vi "Resize Image.vi"(8 "error in (no error)":errorcluster, 11 "Save Image in":refnum<class "Save Image.lvclass">) -> (0 "error out":errorcluster, 3 "Save Image out":refnum<class "Save Image.lvclass">)   [LabVIEW 2018, in "Save Image.lvclass"]
uses:
  Save Image.lvclass
  Interface/Interface.lvclass
  <userlib>/gfitsio/gfitsio.lvlib
  <userlib>/gfitsio/cfitsio-bitpix.ctl
  Simulated_Header/Simulated_Header.lvclass
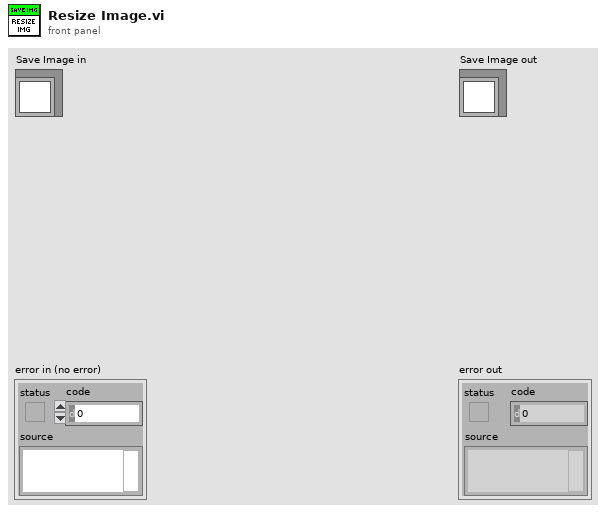
[diagram p1: front panel]
types:
  T1 = typedef "gfitsio.lvlib/cfitsio-bitpix.ctl" = i32
  T2 = cluster{"PREAMP":u16, "READOUT_RATE":u16, "EM_GAIN":u16, "VBIN":u16, "INITIAL_LINE":u16, "INITIAL_COLUMN":u16, "FINAL_LINE":u16, "FINAL_COLUMN":u16, "TRIGGER_MODE":u16, "HBIN":u16, "SHUTTER_TTL":u16, "SHUTTER_MODE":u16, "SHUTTER_OPENING_TIME":u16, "SHUTTER_CLOSING_TIME":u16, "VERTICAL_SHIFT_SPEED":u16, "READ_MODE":u16, "FRAME_TRANSFER":bool, "VERTICAL_CLOCK_VOLTAGE":u16, "ACQUISITION_MODE":u16, "AD_CHANNEL":u16, "EM_MODE":u16}
  T3 = typedef "gfitsio.lvlib/gfitsio-refnum.ctl" = refnum<k1>
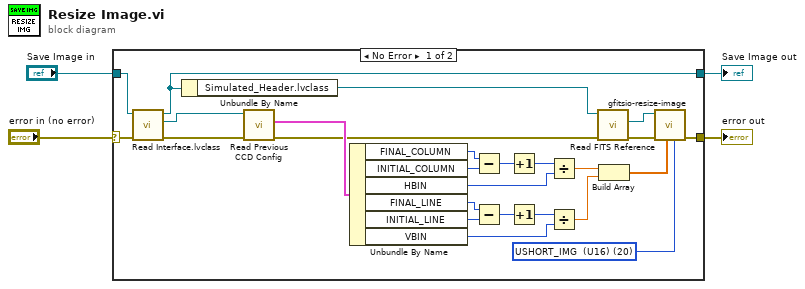
[diagram p0: block diagram]
diagram:
  n1 = case shown="No Error" "error in (no error)" {
    selector: "error in (no error)" -> [w8 w31]
    tunnel: [w12 w31] -> w3
    tunnel: [w5 w30] -> w1
    tunnel: "Save Image in" -> [w9 w30]
    frame No Error {
      w29 = T1 20 items=["<invalid type>"=0, "BYTE_IMG  (U8)"=8, "SHORT_IMG  (I16)"=16, "USHORT_IMG  (U16)"=20, "LONG_IMG  (I32)"=32, "ULONG_IMG  (U32)"=40, "FLOAT_IMG  (SGL)"=-32, "DOUBLE_IMG  (DBL)"=-64] ("image data type")
      n2 = call "Read Interface.lvclass.vi"("error in (no error)"=w8, "Save Image in"=w9) -> ("error out"=w21:errorcluster, "Interface.lvclass"=w20:refnum<class "Interface.lvclass">, "Save Image out"=w5:refnum<class "Save Image.lvclass">)  [unwired: 7 in]
      n3 = Unbundle By Name(w5) -> ("Simulated_Header.lvclass"=w6:refnum<class "Simulated_Header.lvclass">)
      n4 = call "Read Previous CCD Config.vi"("error in (no error)"=w21, "Interface in"=w20) -> ("error out"=w7:errorcluster, "CCD Config"=w28:T2)  [unwired: 7 in, 1 out]
      n5 = Unbundle By Name(w28) -> ("FINAL_COLUMN"=w27:u16, "INITIAL_COLUMN"=w26:u16, "HBIN"=w23:u16, "FINAL_LINE"=w25:u16, "INITIAL_LINE"=w24:u16, "VBIN"=w22:u16)
      n6 = Subtract(x=w27, y=w26) -> (x-y=w16:u16)
      n7 = Subtract(x=w25, y=w24) -> (x-y=w14:u16)
      n8 = Increment(x=w16) -> (x+1=w15:u16)
      n9 = Increment(x=w14) -> (x+1=w13:u16)
      n10 = Divide(x=w15, y=w23) -> (x/y=w19:dbl)
      n11 = Divide(x=w13, y=w22) -> (x/y=w18:dbl)
      n12 = call "Read FITS Reference.vi"("error in (no error)"=w7, "Simulated_Header in"=w6) -> ("error out"=w11:errorcluster, "gfits refnum"=w10:T3)  [unwired: 7 in, 1 out]
      n13 = Build Array(w19, w18) -> (w17:dbl[])
      n14 = call <userlib>:"gfitsio-resize-image.vi"("image data type"=w29, "naxes"=w17, "error in (no error)"=w11, "gfits refnum"=w10) -> ("error out"=w12:errorcluster)  [unwired: 6 in, 1 out]
    }
    frame Error {
    }
  }
  "error out" <- w3
  "Save Image out" <- w1
